vi "NearFiledCamFind.vi"() -> (1 "是否找到相机":bool)   [LabVIEW 2018]
uses:
  <vilib>/vision/driver/NI_Vision_Acquisition_Software.lvlib
panel:
  out "Camera Information Array":T1(array[cluster]) {"BusType" format="%x"; "SerialNumberLow" format="%.0x"; "SerialNumberHigh" format="%.0x"}
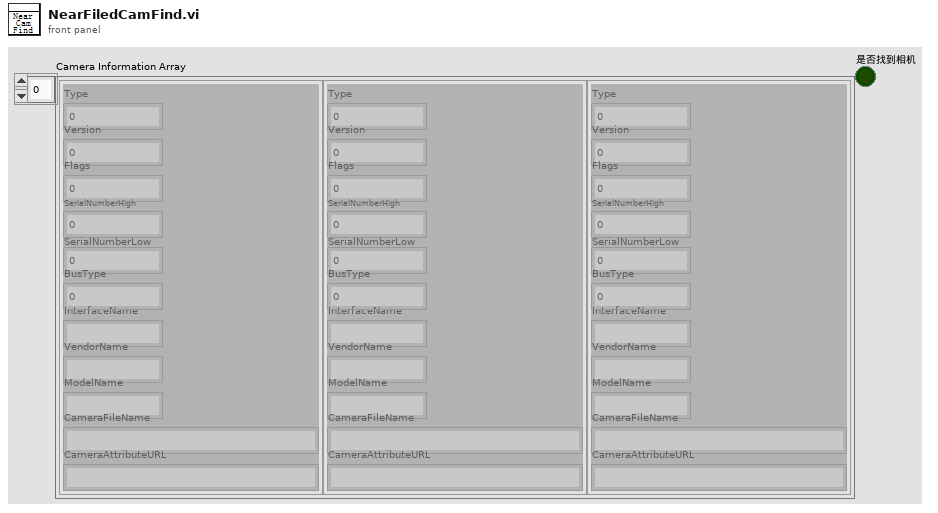
[diagram p1: front panel]
types:
  T1 = cluster{"Type":u32, "Version":u32, "Flags":u32, "SerialNumberHigh":u32, "SerialNumberLow":u32, "BusType":u32, "InterfaceName":string, "VendorName":string, "ModelName":string, "CameraFileName":string, "CameraAttributeURL":string}[]
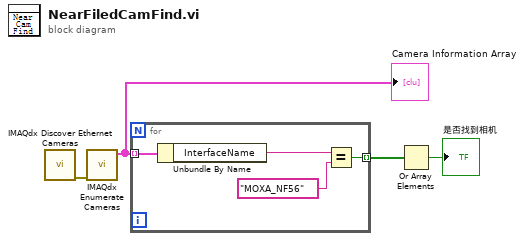
[diagram p0: block diagram]
diagram:
  n1 = call <vilib>:"IMAQdx Discover Ethernet Cameras.vi"() -> ("error out"=w4:errorcluster)  [unwired: 11 in]
  n2 = call <vilib>:"IMAQdx Enumerate Cameras.vi"("error in"=w4) -> ("Camera Information Array"=w3:T1)  [unwired: 9 in, 1 out]
  "Camera Information Array" <- w3
  n3 = for {
    tunnel: w3 -> [w8] mode=indexing
    tunnel: [w5] -> w2 mode=indexing
    n4 = Unbundle By Name(w8) -> ("InterfaceName"=w7:string)
    n5 = Equal?(x=w7, y="MOXA_NF56") -> (x = y?=w5:bool)
  }
  n6 = Or Array Elements(Boolean array=w2) -> (logical OR=→"是否找到相机":bool)
